vi "CWBweather.vi"() -> ()   [LabVIEW 2013]
doc: "This VI reads information from <B>Yahoo! Maps Web Service</B> using DataSocket functions and string parsing. Specifically, this VI reads from this request URL (http://local.yahooapis.com/MapsService/V1/geocode) to pull the latitude and longitude coordinates of the requested location.\n\nNote that this VI works as of Jul 7, 2009 according to the <B>Geocoding API </B>(http://developer.yahoo.com/maps/rest/V1/geocode.html). The following is a detailed description of how the VI retrieves the information from the web service.\n\nBy default, the VI connects to the Web service using Datasocket to retrieve the location of the headquarters of Yahoo:\n\nhttp://local.yahooapis.com/MapsService/V1/geocode?appid=YD-9G7bey8_JXxQP6rxl.fBFGgCdNjoDMACQA--&street=701+First+Ave&city=Sunnyvale&state=CA\n\nwhere <B>701 First Ave, Sunnyvale, CA</B> is the location being queried in this example. The VI then uses string functions to find and parse the latitude and longitude from the text source code returned by Data Socket Read.\n\nThe <B>Street</B>, <B>City</B> and <B>State</B> is concatenated with the root of the Request URL to get the appropriate URL. Data Socket Read returns the Source Code as unformatted text mode. Refer to KB at <B>http://digital.ni.com/public.nsf/allkb/F3CC5F7E60A75CB2862567E700696ABF?OpenDocument</B> for more information on retrieving unformatted text via HTTP using Datasocket. The latitude within this code is listed after the words <Latitude> and before </Latitude>. Match Pattern is used to isolate the coordinates.\n\nThis VI runs in LabVIEW 7.1 onwards."
uses:
  <vilib>/httpClient/LabVIEWHTTPClient.lvlib
panel:
  in  "Tab Control":enum32{"Weather Info", "HtmlString"}(tab)
  out "WeatherTable":string[][](table) caption="今明預報表格"
  out "ReleaseTime":string
  in  "SelectRing":u16(ring) items=["臺北市", "新北市", "臺中市", "臺南市", "高雄市", "基隆市", "桃園縣", "新竹市", "新竹縣", "苗栗縣", "彰化縣", "雲林縣", "嘉義市", "嘉義縣", "屏東縣", "宜蘭縣", "花蓮縣", "臺東縣", "澎湖縣", "金門縣", "連江縣"]
  out "HtmlString":string="<?xml version=\"1.0\"?>\n<ResultSet xmlns:xsi=\"http://www.w3.org/2001/XMLSchema-instance\" xmlns=\"urn:yahoo:maps\" xsi:schemaLocation=\"urn:yahoo:maps http://api.local.yahoo.com/MapsService/V1/GeocodeResponse.xsd\"><Result precision=\"address\"><Latitude>37.416397</Latitude><Longitude>-122.025055</Longitude><Address>701 1st Ave</Address><City>Sunnyvale</City><State>CA</State><Zip>94089-1019</Zip><Country>US</Country></Result></ResultSet>\n<!-- ws04.ydn.gq1.yahoo.com compressed/chunked Mon Apr 13 21:36:32 PDT 2009 -->\n"
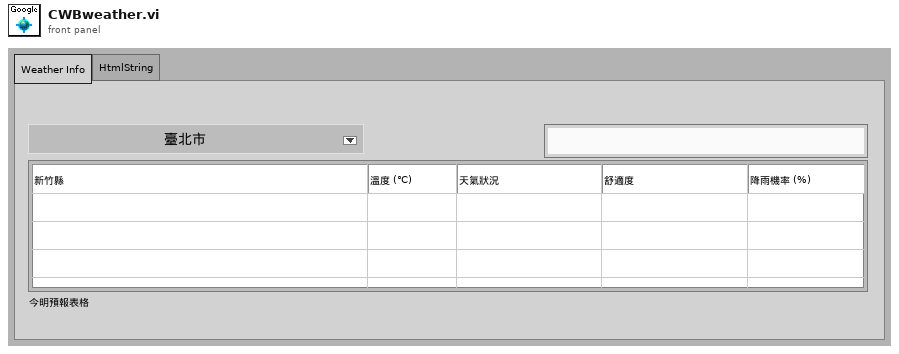
[diagram p1: front panel]
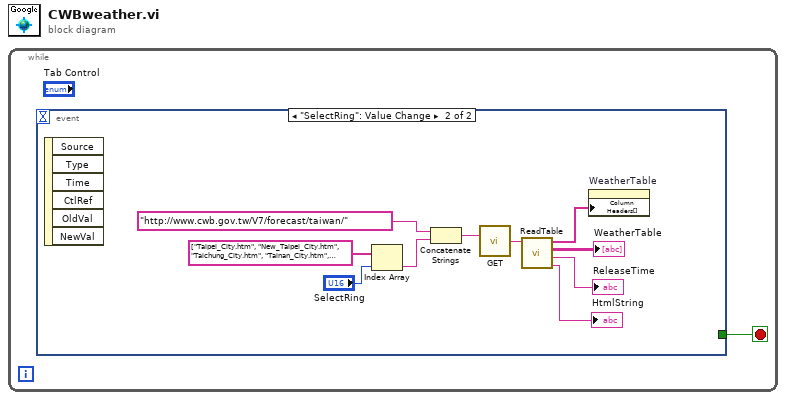
[diagram p0: block diagram]
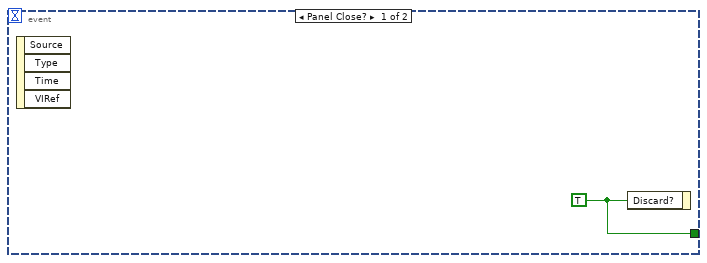
[diagram p2: hidden frame]
diagram:
  n1 = while {
    stop <- w1 stop-if-true
    n2 = event shown="[1] \"SelectRing\": Value Change" {
      selector: _ -> [_ _]
      dyn-events: _ -> [_ _]
      timeout: _ -> [_ _]
      tunnel: [w2 _] -> w1
      event Panel Close? {
        w2 = TRUE ("Discard?")
        n3 = event-data() -> ()  [unwired: 1 in, 4 out]
        n4 = event-data("Discard?"=w2) -> ()  [unwired: 1 in, 1 out]
      }
      event "SelectRing": Value Change {
        n5 = event-data() -> ()  [unwired: 1 in, 6 out]
        n6 = Index Array(array=string[] ["Taipei_City.htm", "New_Taipei_City.htm", "Taichung_City.htm", "Tainan_City.htm", "Kaohsiung_City.htm", "Keelung_City.htm", "Taoyuan_County.htm", "Hsinchu_City.htm", "Hsinchu_County.htm", "Miaoli_County.htm", "Changhua_County.htm", "Yunlin_County.htm", "Chiayi_City.htm", "Chiayi_County.htm", "Pingtung_County.htm", "Yilan_County.htm", "Hualien_County.htm", "Taitung_County.htm", "Penghu_County.htm", "Kinmen_County.htm", "Lienchiang_County.htm"] ("urlString"), index="SelectRing") -> (element=w10:string)
        n7 = Concatenate Strings("http://www.cwb.gov.tw/V7/forecast/taiwan/" ("URL"), w10) -> (w12:string)
        n8 = call <vilib>:"GET.vi"("url"=w12) -> ("body"=w7:string)  [unwired: 11 in, 3 out]
        n9 = call "ReadTable.vi"("HtmlString"=w7) -> ("Big5Text"=→"HtmlString":string, "ReleaseTime"=→"ReleaseTime":string, "tbodyData"=→"WeatherTable":string[][], "theadHead"=w4:string[])  [unwired: 7 in]
        n10 = property on="WeatherTable" class="Tbl (strict)"("Column Headers[]"=w4) -> ()  [unwired: 2 in, 2 out]
      }
    }
  }
